vi "Get Notebooks.vi"(8 "error in (no error)":errorcluster, 11 "Access Token":string) -> (0 "error out":errorcluster, 3 "Response Body":string)   [LabVIEW 2016]
uses:
  Object Oriented Version/Response/Response.lvclass
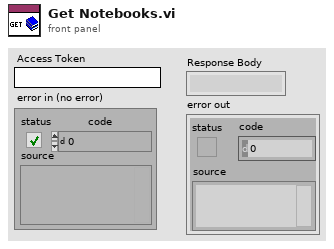
[diagram p1: front panel]
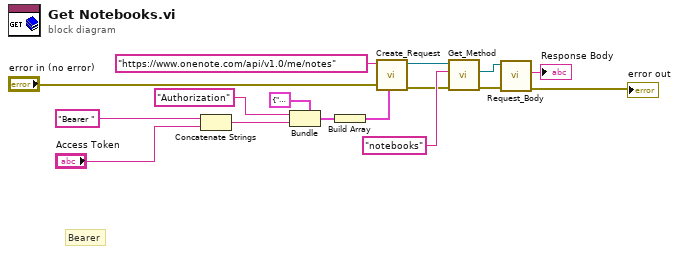
[diagram p0: block diagram]
diagram:
  # "Bearer"
  n1 = Concatenate Strings("Bearer ", "Access Token") -> (w12:string)
  n2 = Bundle(cluster=cluster{"Name":string, "Value":string} {"Name"="", "Value"=""} ("Header"), "Name"="Authorization", "Value"=w12) -> (w10:cluster{"Name":string, "Value":string})
  n3 = Build Array(w10) -> (w14:cluster{"Name":string, "Value":string}[])
  n4 = call "Create_Request.vi"("Headers"=w14, "error in (no error)"="error in (no error)", "Base URL"="https://www.onenote.com/api/v1.0/me/notes") -> ("error out"=w4:errorcluster, "Request out"=w8:refnum<class "Request.lvclass">)  [unwired: 7 in]
  n5 = call "Get_Method.vi"("error in (no error)"=w4, "Endpoint URL"="notebooks", "Request in"=w8) -> ("error out"=w3:errorcluster, "Response out"=w6:refnum<class "Response.lvclass">)  [unwired: 6 in, 1 out]
  n6 = call "Request_Body.vi"("error in (no error)"=w3, "Response in"=w6) -> ("error out"=→"error out":errorcluster, "Response Body"=→"Response Body":string)  [unwired: 7 in, 1 out]
